vi "ClusterDemonstration.vi"() -> ()   [LabVIEW 2018]
panel:
  in  "Cluster":T1 {"Slide 2" scale=0.0..10.0; "Slide 1" scale=0.0..10.0}
  out "Gauge":dbl(knob) scale=0.0..10.0
  # "LabVIEW Cluster Demonstration"
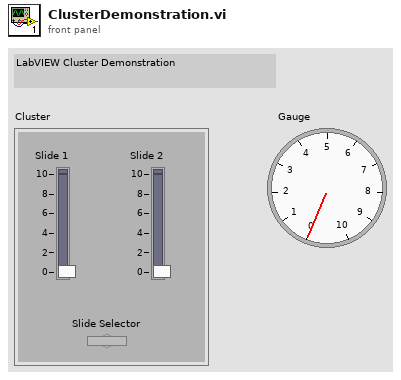
[diagram p1: front panel]
types:
  T1 = cluster{"Slide 1":dbl, "Slide 2":dbl, "Slide Selector":bool}
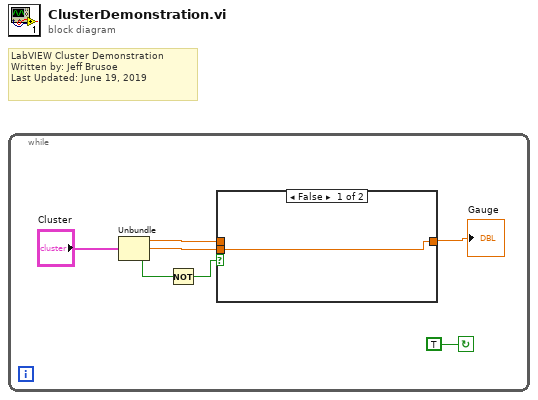
[diagram p0: block diagram]
diagram:
  # "LabVIEW Cluster Demonstration\nWritten by: Jeff Brusoe\nLast Updated: June 19, 2019"
  n1 = while {
    stop <- TRUE continue-if-true
    n2 = Unbundle("Cluster") -> ("Slide 1"=w3:dbl, "Slide 2"=w5:dbl, "Slide Selector"=w2:bool)
    n3 = Not(x=w2) -> (.not. x?=w1:bool)
    n4 = case shown="False" w1 {
      tunnel: w5 -> [w8 _]
      tunnel: [w8 w9] -> w4
      tunnel: w3 -> [_ w9]
      frame False {
      }
      frame True {
      }
    }
    "Gauge" <- w4
  }
